vi "HighEnd-RT.vi"() -> ()   [LabVIEW 2016]
uses:
  GV states.ctl
  Faraday cup states.ctl
  GP307 cluster.ctl
  Glassman Control.ctl
  <vilib>/FPGAPlugInAG/cRIO-9074/niLvFpga_Open_cRIO-9074.vi
  <vilib>/Utility/error.llb/Error Cluster From Error Code.vi
  <vilib>/rvi/errors/niLvFpgaAdjustHostInterfaceError.vi
  <vilib>/rvi/errors/niLvFpgaMergeErrorWithErrorCode.vi
  <vilib>/rvi/interface/nirviOpenFPGA/nirviOpenFPGA.xnode
  Slow-Switching-Control/FPGA Bitfiles/Controlsoftware2_FPGATarget3_HighEnd-FPGA_tW6a4BJhdZw.lvbitx
  HighEnd-FPGA.vi
  <vilib>/rvi/interface/nirviReadWriteControl/nirviReadWriteControl.xnode
  Faraday Cup Readback.ctl
  Gate Valve Readback.ctl
  NiFpgaLv.dll
panel:
  out "Error Reporter":errorcluster
  in  "Tab Control":T1(tab)
  out "ES Quad A+ I readback":fxp<+/-,16,5>
  out "ES Quad A+ V readback":fxp<+/-,16,5>
  out "ES Quad A- I readback":fxp<+/-,16,5>
  out "ES Quad A- V readback":fxp<+/-,16,5>
  out "ES Quad B+ I readback":fxp<+/-,16,5>
  out "Y1- Steerer V set":dbl
  out "Y2+ Steerer V set":dbl
  out "Y2- Steerer V set":dbl
  out "ES Quad A V set":dbl
  out "ES Quad B V set":dbl
  out "ES Quad B+ V readback":fxp<+/-,16,5>
  out "ES Quad B- I readback":fxp<+/-,16,5>
  out "ES Quad B- V readback":fxp<+/-,16,5>
  out "X+ Steerer I readback":fxp<+/-,26,5>
  out "X+ Steerer V readback":fxp<+/-,26,7>
  out "X- Steerer  I readback":fxp<+/-,16,5>
  out "X- Steerer V readback":fxp<+/-,16,5>
  out "Y1+ Steerer  I readback":fxp<+/-,16,5>
  out "Y1+ Steerer V readback":fxp<+/-,16,5>
  out "Y1- Steerer  I readback":fxp<+/-,16,5>
  out "Y1- Steerer V readback":fxp<+/-,16,5>
  out "Y2+ Steerer  I readback":fxp<+/-,16,5>
  out "Y2+ Steerer V readback":fxp<+/-,16,5>
  out "Y2- Steerer  I readback":fxp<+/-,16,5>
  out "Y2- Steerer V readback":fxp<+/-,16,5>
  out "X+ Steerer V set":dbl
  out "X- Steerer V set":dbl
  out "X- Steerer HV Enable":bool
  out "Y1+ Steerer V set":dbl
  out "Y1+ Steerer HV Enable":bool
  out "Y1- Steerer HV Enable":bool
  out "Y2+ Steerer HV Enable":bool
  out "Y2- Steerer HV Enable":bool
  out "ES Quad A HV Enable":bool
  out "ES Quad B HV Enable":bool
  out "X+ Steerer HV Enable":bool
  out "Analyzer Object Vac cluster":T2
  out "Tank Exit Vac cluster":T2
  out "Vac readback loop error":errorcluster
  out "Ion gauge 1":u8[](array[numeric])
  out "Convectron 1":u8[](array[numeric])
  out "Ion gauge 2":u8[](array[numeric])
  out "Convectron 2":u8[](array[numeric])
  out "Ion gauge 3":u8[](array[numeric])
  out "Convectron 4":u8[](array[numeric])
  out "Ion gauge 4":u8[](array[numeric])
  out "Convectron 4":u8[](array[numeric])
  out "High End waist interlock bypass":bool
  out "Tank Exit Vac Interlock":bool
  out "High End Waist Vac Interlock":bool
  out "Analyzer Image Vac Interlock":bool
  out "Tank Exit interlock bypass":bool
  out "Analyzer Image Interlock Bypass":bool
  out "Tank Exit FC Actuator":bool
  out "Cryo Pump GV Actuator":bool
  out "Beamline GV Actuator":bool
  out "Beamline Fast GV actuator":bool
  out "Turbo GV actuator":bool
  out "Beamline Fast GV status":T3
  out "Beamline Fast GV Position":T4
  out "Turbo GV status":T3
  out "Turbo GV Position":T4
  out "Beamline GV status":T3
  out "Beamline GV Position":T4
  out "Tank Exit FC Status":T5
  out "Tank Exit FC Position":cluster{"IN sensor":bool, "OUT sensor":bool}
  out "Cryo Pump GV status":T3
  out "Cryo Pump GV Position":T4
  out "HV readback loop error":errorcluster
  out "Interlock loop error":errorcluster
  out "Actuator Sensor loop error":errorcluster
  out "HV control loop error":errorcluster
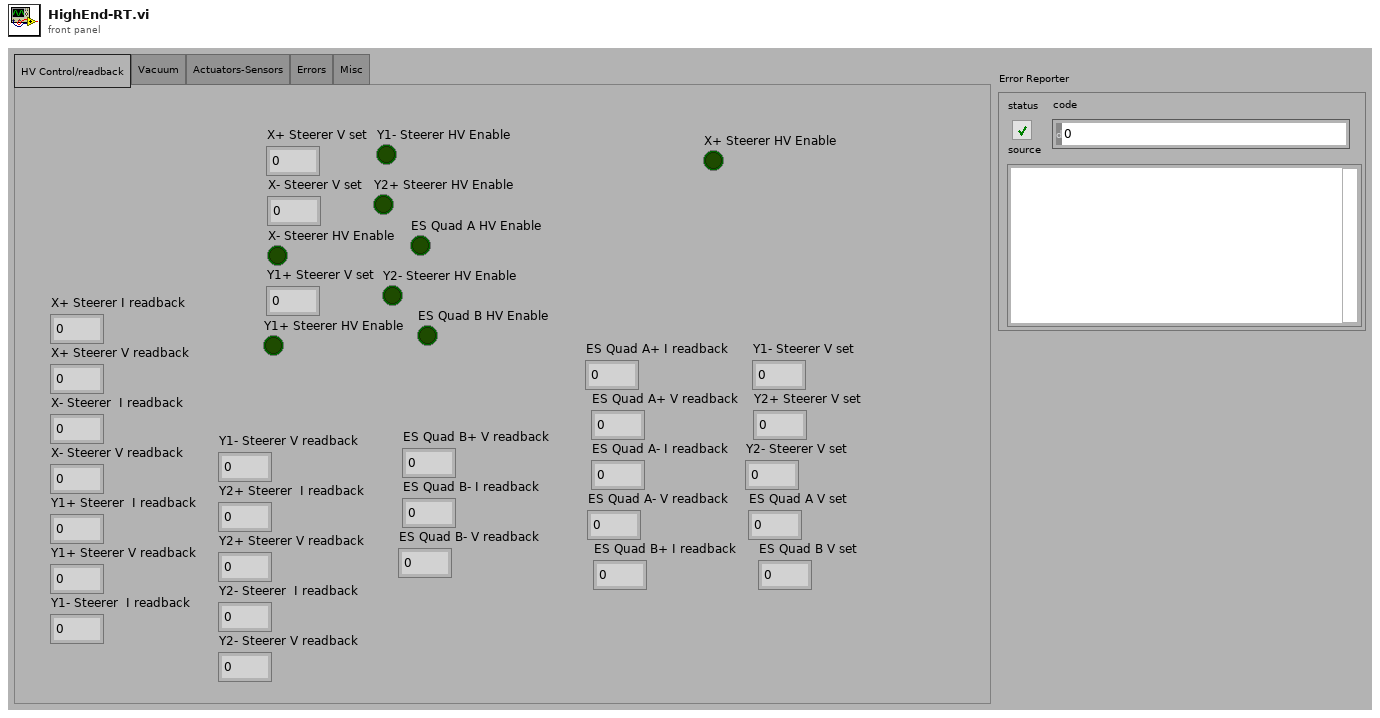
[diagram p1: front panel]
types:
  T1 = enum32{"HV Control/readback", "Vacuum", "Actuators-Sensors", "Errors", "Misc"}
  T2 = cluster{"Ion gauge 1":string, "Convectron  Gauge 1 ":string, "Ion Gauge 2":string, "Convectrom Gauge 2":string}
  T3 = typedef "GV states.ctl" = enum16{"status unclear", "closed", "open"}
  T4 = cluster{"OPEN sensor":bool, "Closed sensor":bool}
  T5 = typedef "Faraday cup states.ctl" = enum16{"FC status unclear", "FC in", "FC out"}
  T6 = typedef "Glassman Control.ctl" = cluster{"V-program":fxp<+/-,16,5>, "HV Enable":bool}
  T7 = typedef "GP307 cluster.ctl" = cluster{"Ion gauge 1":string, "Convectron  Gauge 1 ":string, "Ion Gauge 2":string, "Convectrom Gauge 2":string}
  T8 = typedef "Faraday Cup Readback.ctl" = cluster{"IN sensor":bool, "OUT sensor":bool}
  T9 = typedef "Gate Valve Readback.ctl" = cluster{"OPEN sensor":bool, "Closed sensor":bool}
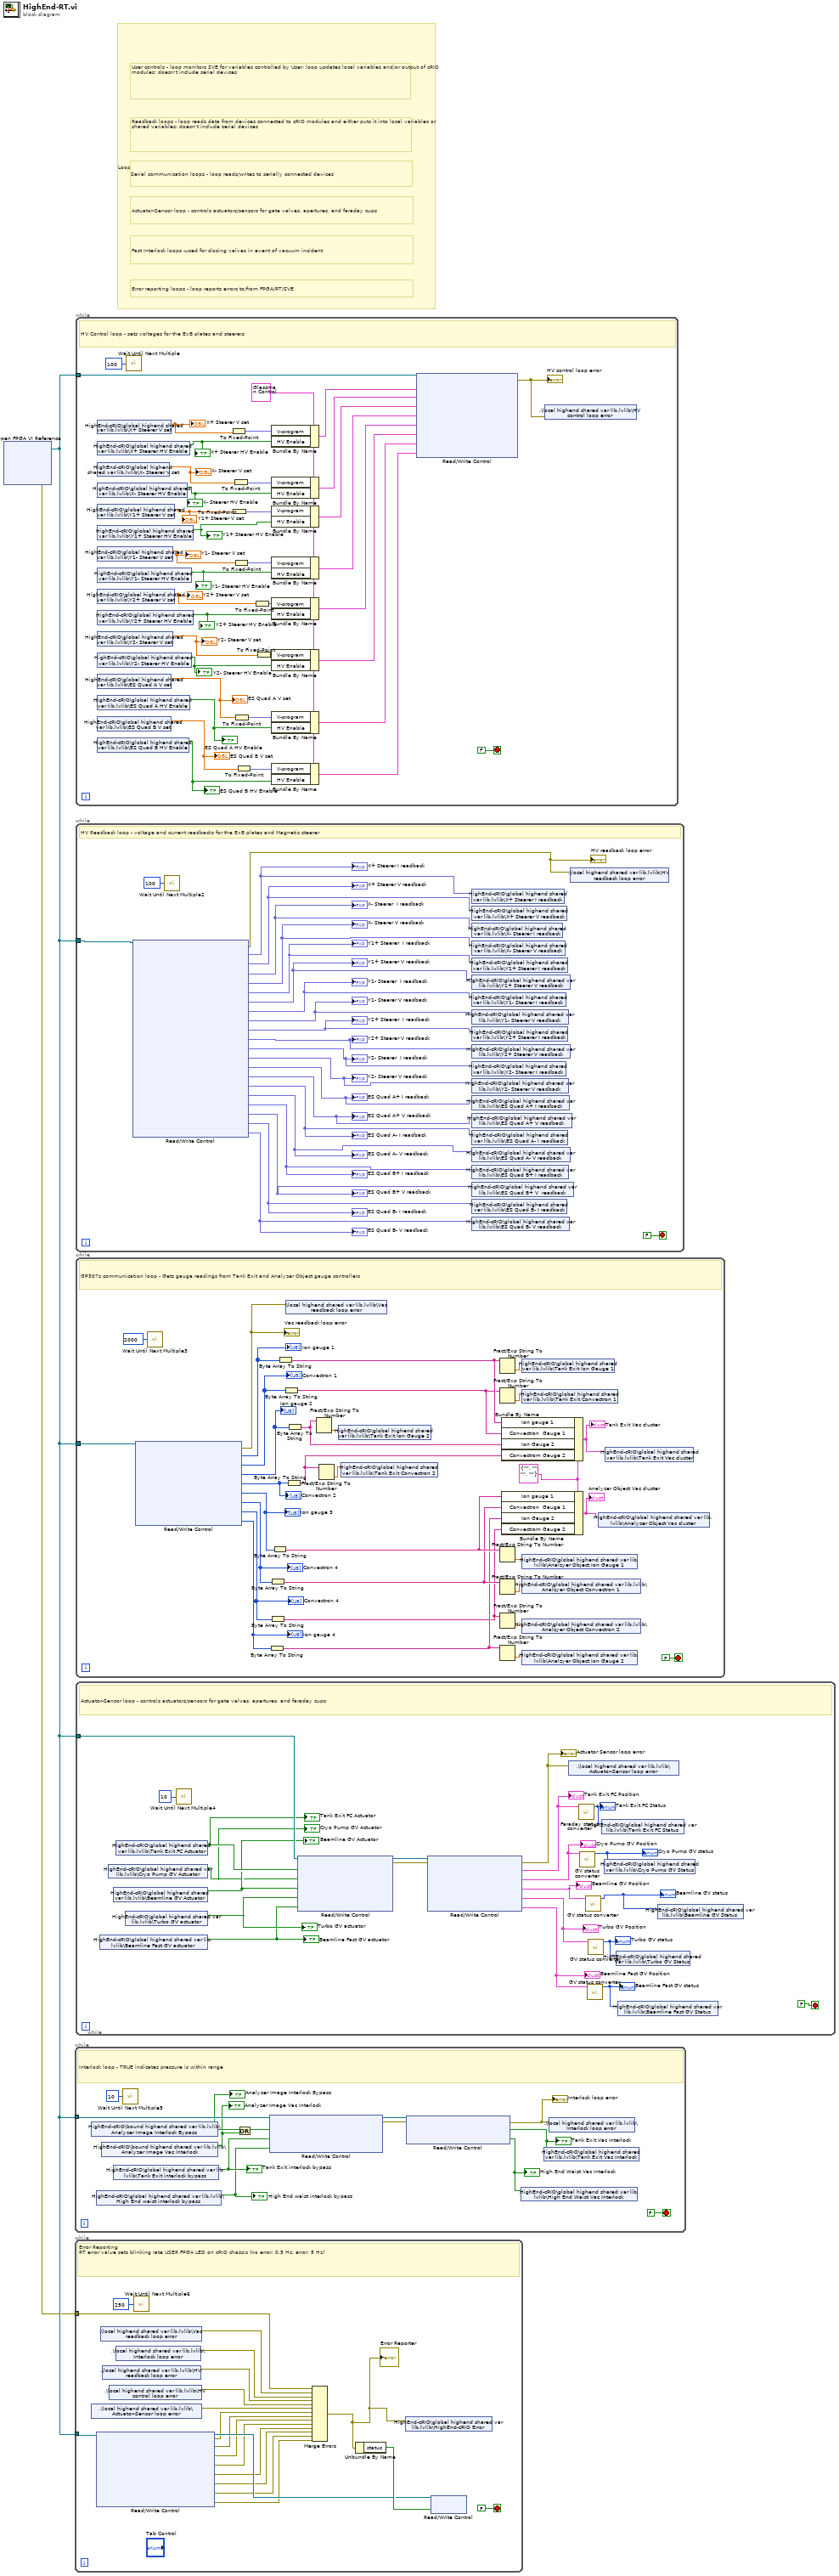
[diagram p0: block diagram]
diagram:
  # "Serial communication loops - loop reads/writes to serially connected devices"
  # "Actuator-Sensor loop - controls actuators/sensors for gate valves, apertures, and faraday cups"
  # "Fast Interlock loops -used for closing valves in event of vacuum incident"
  # "Error reporting loops - loop reports errors to/from FPGA/RT/SVE"
  # "Readback loops - loop reads data from devices connected to cRIO modules and either puts it into local variables or shared variables; doesn't include serial devices"
  # "User controls - loop monitors SVE for variables controlled by User; loop updates local variables and/or output of cRIO modules; doesn't include serial devices"
  # "Loop legend - loops are color coded by responsibility"
  n1 = xnode "Open FPGA VI Reference"() -> ("FPGA VI Reference Out"=w2:refnum<k20>, "error out"=w1:errorcluster)  [unwired: 2 in]
  n2 = while {
    tunnel: w2 -> [w15]
    stop <- FALSE stop-if-true
    # "Interlock loop - TRUE indicates pressure is within range"
    n3 = shared-variable "HighEnd-cRIO\\bound highend shared var lib.lvlib\\Analyzer Image Interlock Bypass"() -> (w11:bool)  [unwired: 1 in, 1 out]
    "Analyzer Image Interlock Bypass" <- w11
    n4 = shared-variable "HighEnd-cRIO\\global highend shared var lib.lvlib\\High End waist interlock bypass"() -> (w6:bool)  [unwired: 1 in, 1 out]
    "High End waist interlock bypass" <- w6
    n5 = shared-variable "HighEnd-cRIO\\bound highend shared var lib.lvlib\\Analyzer Image Vac Interlock"() -> (w9:bool)  [unwired: 1 in, 1 out]
    "Analyzer Image Vac Interlock" <- w9
    n6 = shared-variable "HighEnd-cRIO\\global highend shared var lib.lvlib\\Tank Exit interlock bypass"() -> (w7:bool)  [unwired: 1 in, 1 out]
    "Tank Exit interlock bypass" <- w7
    n7 = call "Wait Until Next Multiple5"("Count(mSec)"=u32 10 ("millisecond multiple")) -> ()  [unwired: 1 out]
    n8 = Or(x=w11, y=w9) -> (x .or. y?=w10:bool)
    n9 = xnode "Read/Write Control"("FPGA VI Reference In"=w15, "Analyzer Image Vac Interlock"=w10, "Tank Exit interlock bypass"=w7, "High End waist interlock bypass"=w6) -> ("FPGA VI Reference Out"=w13:refnum<k20>, "error out"=w12:errorcluster)  [unwired: 1 in]
    n10 = xnode "Read/Write Control"("FPGA VI Reference In"=w13, "error in"=w12) -> ("error out"=w8:errorcluster, "Tank Exit Vac Interlock"=w5:bool, "High End Waist Vac Interlock"=w4:bool)  [unwired: 1 out]
    "Interlock loop error" <- w8
    "Tank Exit Vac Interlock" <- w5
    "High End Waist Vac Interlock" <- w4
    n11 = shared-variable "HighEnd-cRIO\\global highend shared var lib.lvlib\\High End Waist Vac Interlock"(w4) -> ()  [unwired: 1 in, 1 out]
    n12 = shared-variable "HighEnd-cRIO\\global highend shared var lib.lvlib\\Tank Exit Vac Interlock"(w5) -> ()  [unwired: 1 in, 1 out]
    n13 = shared-variable ".\\local highend shared var lib.lvlib\\Interlock loop error"(w8) -> ()  [unwired: 1 in, 1 out]
  }
  n14 = while {
    tunnel: w2 -> [w33]
    tunnel: w1 -> [w17]
    stop <- FALSE stop-if-true
    # "Error Reporting\nRT error value sets blinking rate USER FPGA LED on cRIO chassis (no error: 0.5 Hz; error: 5 Hz)"
    n15 = shared-variable ".\\local highend shared var lib.lvlib\\Actuator-Sensor loop error"() -> (w22:errorcluster)  [unwired: 1 in, 1 out]
    n16 = xnode "Read/Write Control"("FPGA VI Reference In"=w33) -> ("FPGA VI Reference Out"=w32:refnum<k20>, "error out"=w31:errorcluster, "GV Interlock loop error"=w30:errorcluster, "Actuator loop error"=w29:errorcluster, "Tank Exit Vac Gauge error"=w28:errorcluster, "Analyzer Obj Vac Gauge error"=w27:errorcluster, "Steerer HV readback loop error"=w26:errorcluster, "ES Quad HV readback loop error"=w25:errorcluster, "HV control loop error"=w24:errorcluster)  [unwired: 1 in]
    n17 = shared-variable ".\\local highend shared var lib.lvlib\\Vac readback loop error"() -> (w18:errorcluster)  [unwired: 1 in, 1 out]
    n18 = shared-variable ".\\local highend shared var lib.lvlib\\HV readback loop error"() -> (w20:errorcluster)  [unwired: 1 in, 1 out]
    n19 = shared-variable ".\\local highend shared var lib.lvlib\\HV control loop error"() -> (w21:errorcluster)  [unwired: 1 in, 1 out]
    n20 = shared-variable ".\\local highend shared var lib.lvlib\\Interlock loop error"() -> (w19:errorcluster)  [unwired: 1 in, 1 out]
    n21 = call "Wait Until Next Multiple6"("Count(mSec)"=u32 250 ("millisecond multiple")) -> ()  [unwired: 1 out]
    n22 = Merge Errors(w17, w18, w19, w20, w21, w22, w31, w30, w29, w28, w27, w26, w25, w24) -> (w35:errorcluster)
    "Error Reporter" <- w35
    n23 = Unbundle By Name(w35) -> ("status"=w34:bool)
    n24 = shared-variable "HighEnd-cRIO\\global highend shared var lib.lvlib\\HighEnd-cRIO Error"(w35) -> ()  [unwired: 1 in, 1 out]
    n25 = xnode "Read/Write Control"("FPGA VI Reference In"=w32, "RT error"=w34) -> ()  [unwired: 1 in, 2 out]
  }
  n26 = while {
    tunnel: w2 -> [w72]
    stop <- FALSE stop-if-true
    w47 = T6 {"V-program"=0.0, "HV Enable"=FALSE} ("Glassman Control")
    # "HV Control loop - sets voltages for the ExB plates and steerers"
    n27 = shared-variable "HighEnd-cRIO\\global highend shared var lib.lvlib\\X+ Steerer V set"() -> (w68:dbl)  [unwired: 1 in, 1 out]
    "X+ Steerer V set" <- w68
    n28 = shared-variable "HighEnd-cRIO\\global highend shared var lib.lvlib\\X+ Steerer HV Enable"() -> (w67:bool)  [unwired: 1 in, 1 out]
    "X+ Steerer HV Enable" <- w67
    n29 = shared-variable "HighEnd-cRIO\\global highend shared var lib.lvlib\\X- Steerer V set"() -> (w66:dbl)  [unwired: 1 in, 1 out]
    "X- Steerer V set" <- w66
    n30 = shared-variable "HighEnd-cRIO\\global highend shared var lib.lvlib\\X- Steerer HV Enable"() -> (w65:bool)  [unwired: 1 in, 1 out]
    "X- Steerer HV Enable" <- w65
    n31 = shared-variable "HighEnd-cRIO\\global highend shared var lib.lvlib\\Y1+ Steerer V set"() -> (w62:dbl)  [unwired: 1 in, 1 out]
    "Y1+ Steerer V set" <- w62
    n32 = shared-variable "HighEnd-cRIO\\global highend shared var lib.lvlib\\Y1+ Steerer HV Enable"() -> (w39:bool)  [unwired: 1 in, 1 out]
    "Y1+ Steerer HV Enable" <- w39
    n33 = shared-variable "HighEnd-cRIO\\global highend shared var lib.lvlib\\Y1- Steerer V set"() -> (w61:dbl)  [unwired: 1 in, 1 out]
    "Y1- Steerer V set" <- w61
    n34 = shared-variable "HighEnd-cRIO\\global highend shared var lib.lvlib\\Y1- Steerer HV Enable"() -> (w60:bool)  [unwired: 1 in, 1 out]
    "Y1- Steerer HV Enable" <- w60
    n35 = shared-variable "HighEnd-cRIO\\global highend shared var lib.lvlib\\Y2+ Steerer V set"() -> (w57:dbl)  [unwired: 1 in, 1 out]
    "Y2+ Steerer V set" <- w57
    n36 = shared-variable "HighEnd-cRIO\\global highend shared var lib.lvlib\\Y2+ Steerer HV Enable"() -> (w56:bool)  [unwired: 1 in, 1 out]
    "Y2+ Steerer HV Enable" <- w56
    n37 = shared-variable "HighEnd-cRIO\\global highend shared var lib.lvlib\\Y2- Steerer V set"() -> (w55:dbl)  [unwired: 1 in, 1 out]
    "Y2- Steerer V set" <- w55
    n38 = shared-variable "HighEnd-cRIO\\global highend shared var lib.lvlib\\Y2- Steerer HV Enable"() -> (w54:bool)  [unwired: 1 in, 1 out]
    "Y2- Steerer HV Enable" <- w54
    n39 = shared-variable "HighEnd-cRIO\\global highend shared var lib.lvlib\\ES Quad A V set"() -> (w51:dbl)  [unwired: 1 in, 1 out]
    "ES Quad A V set" <- w51
    n40 = shared-variable "HighEnd-cRIO\\global highend shared var lib.lvlib\\ES Quad A HV Enable"() -> (w50:bool)  [unwired: 1 in, 1 out]
    "ES Quad A HV Enable" <- w50
    n41 = shared-variable "HighEnd-cRIO\\global highend shared var lib.lvlib\\ES Quad B V set"() -> (w49:dbl)  [unwired: 1 in, 1 out]
    "ES Quad B V set" <- w49
    n42 = shared-variable "HighEnd-cRIO\\global highend shared var lib.lvlib\\ES Quad B HV Enable"() -> (w48:bool)  [unwired: 1 in, 1 out]
    "ES Quad B HV Enable" <- w48
    n43 = call "Wait Until Next Multiple"("Count(mSec)"=u32 100 ("millisecond multiple")) -> ()  [unwired: 1 out]
    n44 = To Fixed-Point(number=w68) -> (fixed-point=w36:fxp<+/-,16,5>)  [unwired: 1 in]
    n45 = To Fixed-Point(number=w62) -> (fixed-point=w64:fxp<+/-,16,5>)  [unwired: 1 in]
    n46 = To Fixed-Point(number=w66) -> (fixed-point=w70:fxp<+/-,16,5>)  [unwired: 1 in]
    n47 = To Fixed-Point(number=w61) -> (fixed-point=w63:fxp<+/-,16,5>)  [unwired: 1 in]
    n48 = To Fixed-Point(number=w51) -> (fixed-point=w53:fxp<+/-,16,5>)  [unwired: 1 in]
    n49 = To Fixed-Point(number=w49) -> (fixed-point=w52:fxp<+/-,16,5>)  [unwired: 1 in]
    n50 = To Fixed-Point(number=w57) -> (fixed-point=w59:fxp<+/-,16,5>)  [unwired: 1 in]
    n51 = To Fixed-Point(number=w55) -> (fixed-point=w58:fxp<+/-,16,5>)  [unwired: 1 in]
    n52 = Bundle By Name(cluster=w47, "V-program"=w36, "HV Enable"=w67) -> (w71:T6)
    n53 = Bundle By Name(cluster=w47, "V-program"=w70, "HV Enable"=w65) -> (w46:T6)
    n54 = Bundle By Name(cluster=w47, "V-program"=w64, "HV Enable"=w39) -> (w45:T6)
    n55 = Bundle By Name(cluster=w47, "V-program"=w63, "HV Enable"=w60) -> (w44:T6)
    n56 = Bundle By Name(cluster=w47, "V-program"=w59, "HV Enable"=w56) -> (w43:T6)
    n57 = Bundle By Name(cluster=w47, "V-program"=w58, "HV Enable"=w54) -> (w42:T6)
    n58 = Bundle By Name(cluster=w47, "V-program"=w53, "HV Enable"=w50) -> (w41:T6)
    n59 = Bundle By Name(cluster=w47, "V-program"=w52, "HV Enable"=w48) -> (w40:T6)
    n60 = xnode "Read/Write Control"("FPGA VI Reference In"=w72, "X+ Steerer V set"=w71, "X- Steerer V set"=w46, "Y1+ Steerer V set"=w45, "Y1- Steerer V set"=w44, "Y2+ Steerer V set"=w43, "Y2- Steerer V set"=w42, "ES Quad A V set"=w41, "ES Quad B V set"=w40) -> ("error out"=w38:errorcluster)  [unwired: 1 in, 1 out]
    "HV control loop error" <- w38
    n61 = shared-variable ".\\local highend shared var lib.lvlib\\HV control loop error"(error in=w38) -> ()  [unwired: 2 out]
  }
  n62 = while {
    tunnel: w2 -> [w94]
    stop <- FALSE stop-if-true
    # "HV Readback loop - voltage and current readbacks for the ExB plates and Magnetic steerer"
    n63 = xnode "Read/Write Control"("FPGA VI Reference In"=w94) -> ("error out"=w96:errorcluster, "X+ Steerer readback.I-monitor"=w93:fxp<+/-,16,5>, "X+ Steerer readback.V-monitor"=w92:fxp<+/-,16,5>, "X- Steerer readback.I-monitor"=w91:fxp<+/-,16,5>, "X- Steerer readback.V-monitor"=w90:fxp<+/-,16,5>, "Y1+ Steerer readback.I-monitor"=w89:fxp<+/-,16,5>, "Y1+ Steerer readback.V-monitor"=w88:fxp<+/-,16,5>, "Y1- Steerer readback.I-monitor"=w87:fxp<+/-,16,5>, "Y1- Steerer readback.V-monitor"=w86:fxp<+/-,16,5>, "Y2+ Steerer readback.I-monitor"=w85:fxp<+/-,16,5>, "Y2+ Steerer readback.V-monitor"=w84:fxp<+/-,16,5>, "Y2- Steerer readback.I-monitor"=w83:fxp<+/-,16,5>, "Y2- Steerer readback.V-monitor"=w82:fxp<+/-,16,5>, "ES Quad A+ readback.I-monitor"=w81:fxp<+/-,16,5>, "ES Quad A+ readback.V-monitor"=w80:fxp<+/-,16,5>, "ES Quad A- readback.I-monitor"=w74:fxp<+/-,16,5>, "ES Quad A- readback.V-monitor"=w75:fxp<+/-,16,5>, "ES Quad B+ readback.I-monitor"=w76:fxp<+/-,16,5>, "ES Quad B+ readback.V-monitor"=w77:fxp<+/-,16,5>, "ES Quad B- readback.I-monitor"=w78:fxp<+/-,16,5>, "ES Quad B- readback.V-monitor"=w79:fxp<+/-,16,5>)  [unwired: 1 in, 1 out]
    "HV readback loop error" <- w96
    "X+ Steerer I readback" <- w93
    "X+ Steerer V readback" <- w92
    "X- Steerer  I readback" <- w91
    "X- Steerer V readback" <- w90
    "Y1+ Steerer  I readback" <- w89
    "Y1+ Steerer V readback" <- w88
    "Y1- Steerer  I readback" <- w87
    "Y1- Steerer V readback" <- w86
    "Y2+ Steerer  I readback" <- w85
    "Y2+ Steerer V readback" <- w84
    "Y2- Steerer  I readback" <- w83
    "Y2- Steerer V readback" <- w82
    "ES Quad A+ I readback" <- w81
    "ES Quad A+ V readback" <- w80
    "ES Quad A- I readback" <- w74
    "ES Quad A- V readback" <- w75
    "ES Quad B+ I readback" <- w76
    "ES Quad B+ V readback" <- w77
    "ES Quad B- I readback" <- w78
    "ES Quad B- V readback" <- w79
    n64 = call "Wait Until Next Multiple2"("Count(mSec)"=u32 100 ("millisecond multiple")) -> ()  [unwired: 1 out]
    n65 = shared-variable "HighEnd-cRIO\\global highend shared var lib.lvlib\\X+ Steerer I readback"(w93) -> ()  [unwired: 1 in, 1 out]
    n66 = shared-variable "HighEnd-cRIO\\global highend shared var lib.lvlib\\X+ Steerer V readback"(w92) -> ()  [unwired: 1 in, 1 out]
    n67 = shared-variable "HighEnd-cRIO\\global highend shared var lib.lvlib\\X- Steerer I readback"(w91) -> ()  [unwired: 1 in, 1 out]
    n68 = shared-variable "HighEnd-cRIO\\global highend shared var lib.lvlib\\X- Steerer V readback"(w90) -> ()  [unwired: 1 in, 1 out]
    n69 = shared-variable "HighEnd-cRIO\\global highend shared var lib.lvlib\\Y1+ Steerer I readback"(w89) -> ()  [unwired: 1 in, 1 out]
    n70 = shared-variable "HighEnd-cRIO\\global highend shared var lib.lvlib\\Y1+ Steerer V readback"(w88) -> ()  [unwired: 1 in, 1 out]
    n71 = shared-variable "HighEnd-cRIO\\global highend shared var lib.lvlib\\Y1- Steerer I readback"(w87) -> ()  [unwired: 1 in, 1 out]
    n72 = shared-variable "HighEnd-cRIO\\global highend shared var lib.lvlib\\Y1- Steerer V readback"(w86) -> ()  [unwired: 1 in, 1 out]
    n73 = shared-variable "HighEnd-cRIO\\global highend shared var lib.lvlib\\Y2+ Steerer I readback"(w85) -> ()  [unwired: 1 in, 1 out]
    n74 = shared-variable "HighEnd-cRIO\\global highend shared var lib.lvlib\\Y2+ Steerer V readback"(w84) -> ()  [unwired: 1 in, 1 out]
    n75 = shared-variable "HighEnd-cRIO\\global highend shared var lib.lvlib\\Y2- Steerer I readback"(w83) -> ()  [unwired: 1 in, 1 out]
    n76 = shared-variable "HighEnd-cRIO\\global highend shared var lib.lvlib\\Y2- Steerer V readback"(w82) -> ()  [unwired: 1 in, 1 out]
    n77 = shared-variable "HighEnd-cRIO\\global highend shared var lib.lvlib\\ES Quad A+ I readback"(w81) -> ()  [unwired: 1 in, 1 out]
    n78 = shared-variable "HighEnd-cRIO\\global highend shared var lib.lvlib\\ES Quad A+ V readback"(w80) -> ()  [unwired: 1 in, 1 out]
    n79 = shared-variable "HighEnd-cRIO\\global highend shared var lib.lvlib\\ES Quad A- I readback"(w74) -> ()  [unwired: 1 in, 1 out]
    n80 = shared-variable "HighEnd-cRIO\\global highend shared var lib.lvlib\\ES Quad A- V readback"(w75) -> ()  [unwired: 1 in, 1 out]
    n81 = shared-variable "HighEnd-cRIO\\global highend shared var lib.lvlib\\ES Quad B+ I readback"(w76) -> ()  [unwired: 1 in, 1 out]
    n82 = shared-variable "HighEnd-cRIO\\global highend shared var lib.lvlib\\ES Quad B+ V  readback"(w77) -> ()  [unwired: 1 in, 1 out]
    n83 = shared-variable "HighEnd-cRIO\\global highend shared var lib.lvlib\\ES Quad B- I readback"(w78) -> ()  [unwired: 1 in, 1 out]
    n84 = shared-variable "HighEnd-cRIO\\global highend shared var lib.lvlib\\ES Quad B- V readback"(w79) -> ()  [unwired: 1 in, 1 out]
    n85 = shared-variable ".\\local highend shared var lib.lvlib\\HV readback loop error"(w96) -> ()  [unwired: 1 in, 1 out]
  }
  n86 = while {
    tunnel: w2 -> [w109]
    stop <- FALSE stop-if-true
    w108 = T7 {"Ion gauge 1"="", "Convectron  Gauge 1 "="", "Ion Gauge 2"="", "Convectrom Gauge 2"=""} ("Ion gauge cluster control")
    # "GP307s communication loop - Gets gauge readings from Tank Exit and Analyzer Object gauge controllers"
    n87 = xnode "Read/Write Control"("FPGA VI Reference In"=w109) -> ("error out"=w107:errorcluster, "Tank Exit Ion Gauge 1"=w124:u8[], "Tank Exit Convectron 1"=w125:u8[], "Tank Exit Ion Gauge 2"=w126:u8[], "Tank Exit Convectron 2"=w127:u8[], "Analyzer Object Ion Gauge 1"=w122:u8[], "Analyzer Object Convectron 1"=w121:u8[], "Analyzer Object Convectron 2"=w119:u8[], "Analyzer Object Ion Gauge 2"=w120:u8[])  [unwired: 1 in, 1 out]
    "Vac readback loop error" <- w107
    "Ion gauge 1" <- w124
    "Convectron 1" <- w125
    "Ion gauge 2" <- w126
    "Convectron 2" <- w127
    "Ion gauge 3" <- w122
    "Convectron 4" <- w121
    "Ion gauge 4" <- w120
    "Convectron 4" <- w119
    n88 = call "Wait Until Next Multiple3"("Count(mSec)"=u32 2000 ("millisecond multiple")) -> ()  [unwired: 1 out]
    n89 = Byte Array To String(unsigned byte array=w120) -> (string=w115:string)
    n90 = Byte Array To String(unsigned byte array=w121) -> (string=w116:string)
    n91 = Byte Array To String(unsigned byte array=w119) -> (string=w114:string)
    n92 = Byte Array To String(unsigned byte array=w122) -> (string=w117:string)
    n93 = Byte Array To String(unsigned byte array=w124) -> (string=w113:string)
    n94 = Byte Array To String(unsigned byte array=w125) -> (string=w112:string)
    n95 = shared-variable ".\\local highend shared var lib.lvlib\\Vac readback loop error"(w107) -> ()  [unwired: 1 in, 1 out]
    n96 = Byte Array To String(unsigned byte array=w127) -> (string=w110:string)
    n97 = Byte Array To String(unsigned byte array=w126) -> (string=w111:string)
    n98 = Fract/Exp String To Number(string=w111) -> (number=w106:dbl)  [unwired: 3 in, 1 out]
    n99 = Fract/Exp String To Number(string=w110) -> (number=w105:dbl)  [unwired: 3 in, 1 out]
    n100 = shared-variable "HighEnd-cRIO\\global highend shared var lib.lvlib\\Tank Exit Ion Gauge 2"(w106) -> ()  [unwired: 1 in, 1 out]
    n101 = shared-variable "HighEnd-cRIO\\global highend shared var lib.lvlib\\Tank Exit Convectron 2"(w105) -> ()  [unwired: 1 in, 1 out]
    n102 = Fract/Exp String To Number(string=w113) -> (number=w104:dbl)  [unwired: 3 in, 1 out]
    n103 = Fract/Exp String To Number(string=w112) -> (number=w103:dbl)  [unwired: 3 in, 1 out]
    n104 = Fract/Exp String To Number(string=w117) -> (number=w102:dbl)  [unwired: 3 in, 1 out]
    n105 = Fract/Exp String To Number(string=w116) -> (number=w101:dbl)  [unwired: 3 in, 1 out]
    n106 = Fract/Exp String To Number(string=w114) -> (number=w100:dbl)  [unwired: 3 in, 1 out]
    n107 = Fract/Exp String To Number(string=w115) -> (number=w99:dbl)  [unwired: 3 in, 1 out]
    n108 = Bundle By Name(cluster=w108, "Ion gauge 1"=w113, "Convectron  Gauge 1"=w112, "Ion Gauge 2"=w111, "Convectrom Gauge 2"=w110) -> (w118:T7)
    "Tank Exit Vac cluster" <- w118
    n109 = Bundle By Name(cluster=w108, "Ion gauge 1"=w117, "Convectron  Gauge 1"=w116, "Ion Gauge 2"=w115, "Convectrom Gauge 2"=w114) -> (w98:T7)
    "Analyzer Object Vac cluster" <- w98
    n110 = shared-variable "HighEnd-cRIO\\global highend shared var lib.lvlib\\Tank Exit Ion Gauge 1"(w104) -> ()  [unwired: 1 in, 1 out]
    n111 = shared-variable "HighEnd-cRIO\\global highend shared var lib.lvlib\\Tank Exit Convectron 1"(w103) -> ()  [unwired: 1 in, 1 out]
    n112 = shared-variable "HighEnd-cRIO\\global highend shared var lib.lvlib\\Analzyer Object Ion Gauge 1"(w102) -> ()  [unwired: 1 in, 1 out]
    n113 = shared-variable "HighEnd-cRIO\\global highend shared var lib.lvlib\\Analzyer Object Convectron 1"(w101) -> ()  [unwired: 1 in, 1 out]
    n114 = shared-variable "HighEnd-cRIO\\global highend shared var lib.lvlib\\Analzyer Object Convectron 2"(w100) -> ()  [unwired: 1 in, 1 out]
    n115 = shared-variable "HighEnd-cRIO\\global highend shared var lib.lvlib\\Analzyer Object Ion Gauge 2"(w99) -> ()  [unwired: 1 in, 1 out]
    n116 = shared-variable "HighEnd-cRIO\\global highend shared var lib.lvlib\\Analyzer Object Vac cluster"(w98) -> ()  [unwired: 1 in, 1 out]
    n117 = shared-variable "HighEnd-cRIO\\global highend shared var lib.lvlib\\Tank Exit Vac cluster"(w118) -> ()  [unwired: 1 in, 1 out]
  }
  n118 = while {
    tunnel: w2 -> [w138]
    stop <- FALSE stop-if-true
    # "Actuator-Sensor loop - controls actuators/sensors for gate valves, apertures, and faraday cups"
    n119 = shared-variable "HighEnd-cRIO\\global highend shared var lib.lvlib\\Beamline Fast GV actuator"() -> (w134:bool)  [unwired: 1 in, 1 out]
    "Beamline Fast GV actuator" <- w134
    n120 = shared-variable "HighEnd-cRIO\\global highend shared var lib.lvlib\\Cryo Pump GV Actuator"() -> (w133:bool)  [unwired: 1 in, 1 out]
    "Cryo Pump GV Actuator" <- w133
    n121 = shared-variable "HighEnd-cRIO\\global highend shared var lib.lvlib\\Beamline GV Actuator"() -> (w136:bool)  [unwired: 1 in, 1 out]
    "Beamline GV Actuator" <- w136
    n122 = shared-variable "HighEnd-cRIO\\global highend shared var lib.lvlib\\Tank Exit FC Actuator"() -> (w137:bool)  [unwired: 1 in, 1 out]
    "Tank Exit FC Actuator" <- w137
    n123 = shared-variable "HighEnd-cRIO\\global highend shared var lib.lvlib\\Turbo GV actuator"() -> (w135:bool)  [unwired: 1 in, 1 out]
    "Turbo GV actuator" <- w135
    n124 = call "Wait Until Next Multiple4"("Count(mSec)"=u32 10 ("millisecond multiple")) -> ()  [unwired: 1 out]
    n125 = xnode "Read/Write Control"("FPGA VI Reference In"=w138, "Tank Exit FC Actuator"=w137, "Cryo Pump GV Actuator"=w133, "Beamline GV Actuator"=w136, "Turbo GV actuator"=w135, "Beamline Fast GV actuator"=w134) -> ("FPGA VI Reference Out"=w147:refnum<k20>, "error out"=w146:errorcluster)  [unwired: 1 in]
    n126 = xnode "Read/Write Control"("FPGA VI Reference In"=w147, "error in"=w146) -> ("error out"=w132:errorcluster, "Tank Exit FC Position"=w142:T8, "Cryo Pump GV Position"=w139:T9, "Beamline GV Position"=w144:T9, "Turbo GV Position"=w141:T9, "Beamline Fast GV Position"=w143:T9)  [unwired: 1 out]
    "Actuator Sensor loop error" <- w132
    "Cryo Pump GV Position" <- w139
    "Tank Exit FC Position" <- w142
    "Beamline GV Position" <- w144
    "Turbo GV Position" <- w141
    "Beamline Fast GV Position" <- w143
    n127 = shared-variable ".\\local highend shared var lib.lvlib\\Actuator-Sensor loop error"(w132) -> ()  [unwired: 1 in, 1 out]
    n128 = call "Faraday status converter.vi"("FC Position"=w142) -> ("FC Status"=w145:T5)  [unwired: 10 in]
    "Tank Exit FC Status" <- w145
    n129 = call "GV status converter.vi"("Gate Valve"=w139) -> ("GV Status"=w140:T3)  [unwired: 10 in]
    "Cryo Pump GV status" <- w140
    n130 = call "GV status converter.vi"("Gate Valve"=w144) -> ("GV Status"=w129:T3)  [unwired: 10 in]
    "Beamline GV status" <- w129
    n131 = call "GV status converter.vi"("Gate Valve"=w143) -> ("GV Status"=w131:T3)  [unwired: 10 in]
    "Beamline Fast GV status" <- w131
    n132 = call "GV status converter.vi"("Gate Valve"=w141) -> ("GV Status"=w130:T3)  [unwired: 10 in]
    "Turbo GV status" <- w130
    n133 = shared-variable "HighEnd-cRIO\\global highend shared var lib.lvlib\\Tank Exit FC Status"(w145) -> ()  [unwired: 1 in, 1 out]
    n134 = shared-variable "HighEnd-cRIO\\global highend shared var lib.lvlib\\Cryo Pump GV Status"(w140) -> ()  [unwired: 1 in, 1 out]
    n135 = shared-variable "HighEnd-cRIO\\global highend shared var lib.lvlib\\Turbo GV Status"(w130) -> ()  [unwired: 1 in, 1 out]
    n136 = shared-variable "HighEnd-cRIO\\global highend shared var lib.lvlib\\Beamline Fast GV Status"(w131) -> ()  [unwired: 1 in, 1 out]
    n137 = shared-variable "HighEnd-cRIO\\global highend shared var lib.lvlib\\Beamline GV Status"(w129) -> ()  [unwired: 1 in, 1 out]
  }
